vi "GitGetAllAuthors.vi"(8 "error in (no error)":errorcluster, 9 "Directory":path=path "", 11 "Git exec":string="git") -> (0 "error out":errorcluster, 1 "Directory out":path, 2 "Author Array":string[](array[string]), 3 "Git exec out":string="git")   [LabVIEW 2013]
uses:
  <vilib>/Utility/error.llb/whitespace.ctl
  GitCmd.vi
  <vilib>/dlg_ctls.llb/Space Constant.vi
  GitUtils/PathtoDirPath.vi
  <vilib>/Platform/system.llb/System Exec.vi
  <vilib>/Utility/error.llb/Error Cluster From Error Code.vi
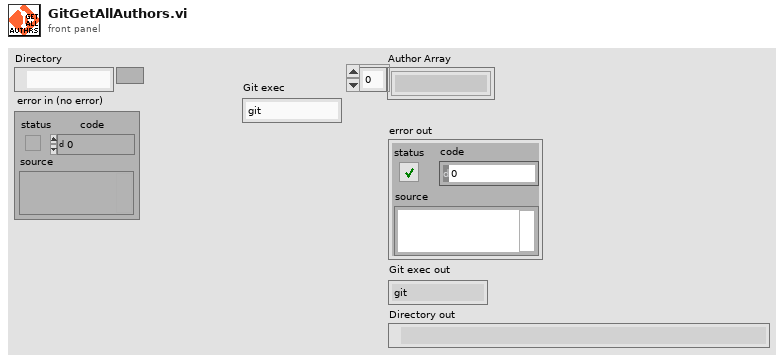
[diagram p1: front panel]
types:
  T1 = typedef "whitespace.ctl" = u16
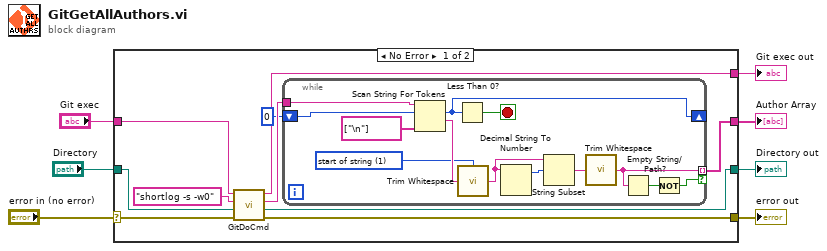
[diagram p0: block diagram]
diagram:
  n1 = case shown="No Error" "error in (no error)" {
    selector: "error in (no error)" -> [w13 w33]
    tunnel: "Git exec" -> [w11 w31]
    tunnel: "Directory" -> [w12 w32]
    tunnel: [w9 _] -> w1
    tunnel: [w17 w33] -> w5
    tunnel: [w16 w32] -> w3
    tunnel: [w15 w31] -> w2
    frame No Error {
      n2 = call "GitDoCmd.vi"("error in (no error)"=w13, "Working Path"=w12, "Git command"="shortlog -s -w0" ("string"), "Git exec"=w11) -> ("error out"=w17:errorcluster, "Working Path out"=w16:path, "Returned stdout"=w10:string, "Git exec out"=w15:string)  [unwired: 3 in]
      n3 = while {
        shift-right: [w28] -> _
        shift-left: 0 ("offset past token") -> [w30]
        tunnel: w10 -> [w26]
        tunnel: [w19] -> w9 mode=indexing if=w24
        stop <- w27 stop-if-true
        w18 = T1 1 items=["both", "start of string", "end of string"] ("location (both)")
        n4 = Scan String For Tokens(6:string[] ["\n"] ("delimiters (\\s,\\t,\\r,\\n)"), 8:w30, 9:w26) -> (1:w21:string, 2:w28:i32)  [unwired: 3 in, 2 out]
        n5 = Less Than 0?(x=w28) -> (x < 0?=w27:bool)
        n6 = call <vilib>:"Trim Whitespace.vi"("string"=w21, "location (both)"=w18) -> ("trimmed string"=w22:string)
        n7 = Decimal String To Number(string=w22) -> (offset past number=w25:i32)  [unwired: 2 in, 1 out]
        n8 = String Subset(string=w22, offset (0)=w25) -> (substring=w20:string)  [unwired: 1 in]
        n9 = call <vilib>:"Trim Whitespace.vi"("string"=w20) -> ("trimmed string"=w19:string)  [unwired: 1 in]
        n10 = Empty String/Path?(string/path=w19) -> (empty?=w23:bool)
        n11 = Not(x=w23) -> (.not. x?=w24:bool)
      }
    }
    frame Error {
    }
  }
  "error out" <- w5
  "Git exec out" <- w2
  "Directory out" <- w3
  "Author Array" <- w1
